vi "LEBITplc.PubSetValueInfo.vi"(0 "i ref in":refnum<vi>, 2 "i attribute in":T1, 5 "error in":errorcluster) -> (14 "i ref out":refnum<vi>, 16 "i attribute out":T1, 17 "SetValueInfoServiceID":i32[](array[numeric]), 19 "error out":errorcluster)   [LabVIEW 2014, in "LEBITplc.lvlib"]
uses:
  LEBITplc.lvlib
  LEBITplc.i attribute.ctl
  CSlibraries/UtilityLib/UtilityLib.valueStatus.ctl
  CSlibraries/UtilityLib/UtilityLib.lvlib
  CS_Core/CSSystem/CoreLib/CoreLib.lvlib
  CSlibraries-extern/DimLVEvent/LVDimInterface/LVDimInterface.lvlib
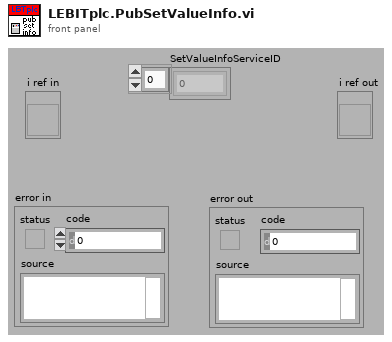
[diagram p1: front panel]
types:
  T1 = typedef "LEBITplc.lvlib/LEBITplc.i attribute.ctl" = cluster{"LLFLocation":string, "SetFileLocation":string, "nickNames":string[], "setValuePLCServiceID":i32[], "GUIServiceID":i32[], "monValuePLC":string[], "SetValueServiceID":i32[], "MonValueServiceID":i32[], "SetValue":dbl[][], "SetValueMin":dbl[], "SetValueMax":dbl[], "SetValueInfoServiceID":i32[], "GUINames":string[], "ListOfBases":string[], "Scale":dbl[], "Offset":dbl[], "setValuePLC":string[], "BaseName":string[], "ScaleServiceID":i32[], "OffsetServiceID":i32[], "AllPLCValues":string[], "CondSpecialArray":string[][], "CondSpecialIndex":i32[], "CondSpecialMonValue":dbl[], "RecentlyChanged":i32[], "SetFileLocationID":i32, "Dependent-Monitors":string[][], "LastLoadedFiles":string[], "IonGuideCalibLocation":string, "Monitor Dependent":string[], "Special":string[], "PLC?":bool[], "Start Date":string, "ListOfBasesServiceID":i32, "SETRA VISA resource":refnum<visa-resource-name>}
  T2 = typedef "UtilityLib.lvlib/UtilityLib.valueStatus.ctl" = enum16{"no info available", "stand by/off", "on", "warning", "alarm/malfunction", "not implemented", "user action required", "important information", "system default", "control default", "indicator default", "button default"}
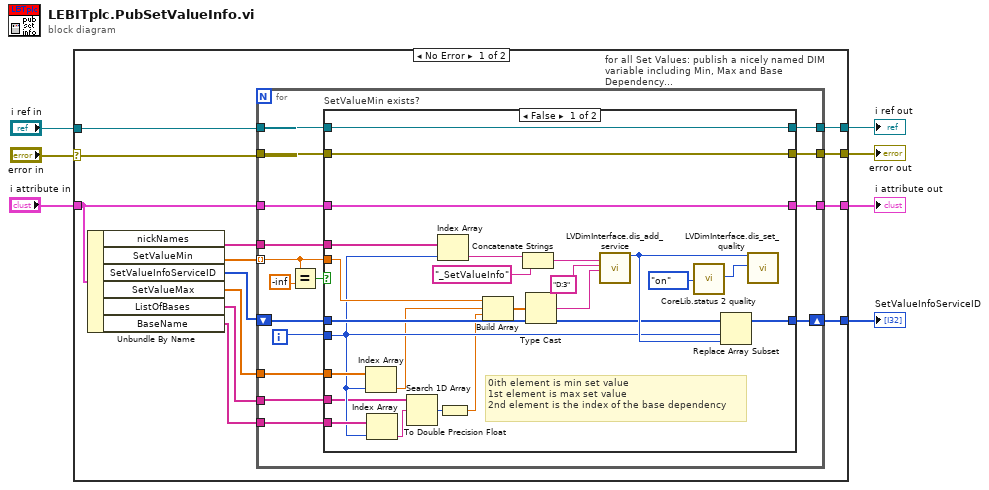
[diagram p0: block diagram]
diagram:
  n1 = case shown="No Error" "error in" {
    selector: "error in" -> [w11 w66]
    tunnel: "i attribute in" -> [w9 w65]
    tunnel: [w20 w66] -> w6
    tunnel: [w19 w67] -> w5
    tunnel: "i ref in" -> [w17 w67]
    tunnel: [w13 _] -> w3
    tunnel: [w8 w65] -> w1
    frame No Error {
      n2 = Unbundle By Name(w9) -> ("nickNames"=w16:string[], "SetValueMin"=w18:dbl[], "SetValueInfoServiceID"=w14:i32[], "SetValueMax"=w15:dbl[], "ListOfBases"=w10:string[], "BaseName"=w12:string[])
      n3 = for "for all Set Values: publish a nicely named DIM variable including Min, Max and Base Dependency..." {
        tunnel: w16 -> [w30]
        tunnel: w18 -> [w27] mode=indexing
        tunnel: w17 -> [w34]
        tunnel: w11 -> [w33]
        tunnel: [w31] -> w20
        tunnel: [w32] -> w19
        shift-right: [w26] -> w13
        shift-left: w14 -> [w35]
        tunnel: w15 -> [w25]
        tunnel: w10 -> [w23]
        tunnel: w12 -> [w24]
        tunnel: w9 -> [w22]
        tunnel: [w21] -> w8
        i -> [w36]
        n4 = Equal?(x=w27, y=-inf) -> (x = y?=w29:bool)
        n5 = case "SetValueMin exists?" shown="False" w29 {
          tunnel: w36 -> [w43 _]
          tunnel: w35 -> [w51 w62]
          tunnel: w34 -> [w55 w64]
          tunnel: w33 -> [w54 w63]
          tunnel: [w55 w64] -> w32
          tunnel: [w54 w63] -> w31
          tunnel: w30 -> [w48 _]
          tunnel: w27 -> [w45 _]
          tunnel: [w50 w62] -> w26
          tunnel: w25 -> [w49 _]
          tunnel: w24 -> [w44 _]
          tunnel: w23 -> [w41 _]
          tunnel: w22 -> [w37 w61]
          tunnel: [w37 w61] -> w21
          frame False {
            # "0ith element is min set value\n1st element is max set value\n2nd element is the index of the base dependency"
            n6 = Index Array(array=w49, index=w43) -> (element=w42:dbl)
            n7 = Index Array(array=w44, index=w43) -> (element=w40:string)
            n8 = Search 1D Array(1D array=w41, element=w40) -> (index of element=w38:i32)  [unwired: 1 in]
            n9 = Index Array(array=w48, index=w43) -> (element=w47:string)
            n10 = To Double Precision Float(number=w38) -> (double precision float=w39:dbl)
            n11 = Build Array(w45, w42, w39) -> (w46:dbl[])
            n12 = Concatenate Strings(w47, "_SetValueInfo" ("string")) -> (w59:string)
            n13 = Type Cast(x=w46) -> (*(type *) &x=w52:string)  [unwired: 1 in]
            n14 = call "LVDimInterface.dis_add_service.vi"("serviceName"=w59, "typeDescriptor"="D:3", "data"=w52) -> ("my_serviceID"=w56:i32)  [unwired: 15 in, 1 out]
            n15 = call "CoreLib.status 2 quality.vi"("valueStatus"=UtilityLib.valueStatus."on") -> ("quality"=w58:i32)  [unwired: 18 in]
            n16 = Replace Array Subset(array=w51, new element=w56, index=w43) -> (w50:i32[])
            n17 = call "LVDimInterface.dis_set_quality.vi"("my_serviceID"=w56, "quality"=w58) -> ()  [unwired: 16 in, 2 out]
          }
          frame True {
          }
        }
      }
    }
    frame Error {
    }
  }
  "error out" <- w6
  "i ref out" <- w5
  "SetValueInfoServiceID" <- w3
  "i attribute out" <- w1
